vi "실습 4-1 배열 만들기(컨트롤배열).vi"() -> ()   [LabVIEW 2014]
panel:
  out "x+y":dbl[][](array[numeric])
  in  "배열":dbl[][](array[numeric])
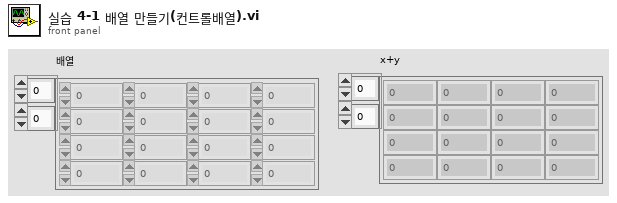
[diagram p1: front panel]
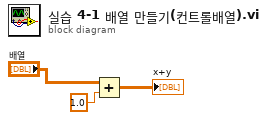
[diagram p0: block diagram]
diagram:
  n1 = Add(x="배열", y=1.0) -> (x+y=→"x+y":dbl[][])
